vi "Get image names in directory.vi"(8 "error in (no error)":errorcluster, 10 "Image Path":string, 11 "Interface in":refnum<class "Interface.lvclass">) -> (0 "error out":errorcluster, 3 "Interface out":refnum<class "Interface.lvclass">)   [LabVIEW 2018, in "Interface.lvclass"]
uses:
  Interface.lvclass
  Interface.lvclass/Interface.ctl
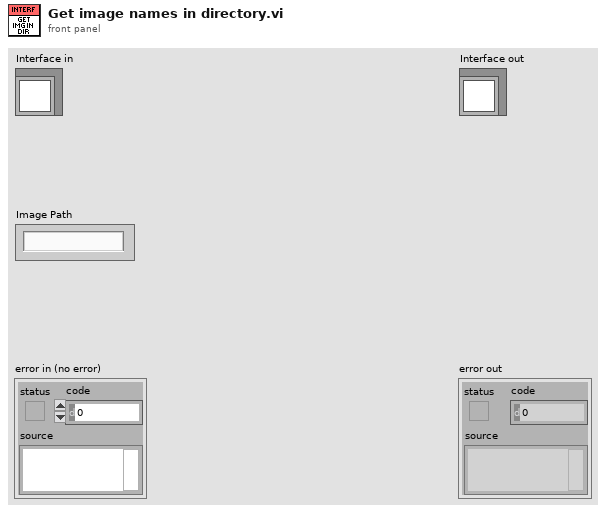
[diagram p1: front panel]
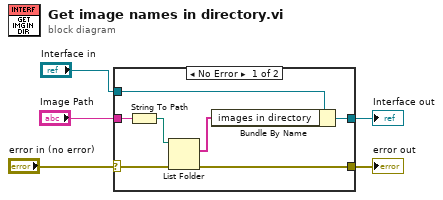
[diagram p0: block diagram]
diagram:
  n1 = case shown="No Error" "error in (no error)" {
    selector: "error in (no error)" -> [w11 w14]
    tunnel: [w10 w14] -> w4
    tunnel: "Image Path" -> [w9 _]
    tunnel: "Interface in" -> [w8 w13]
    tunnel: [w7 w13] -> w1
    frame No Error {
      n2 = String To Path(string=w9) -> (path=w12:path)
      n3 = List Folder(path=w12, error in=w11) -> (filenames=w6:string[], error out=w10:errorcluster)  [unwired: 2 in, 2 out]
      n4 = Bundle By Name(cluster=w8, "images in directory"=w6) -> (w7:refnum<class "Interface.lvclass">)
    }
    frame Error {
    }
  }
  "error out" <- w4
  "Interface out" <- w1
